vi "Write Config Files.vi"(8 "error in (no error)":errorcluster, 10 "Accessors:Config Session":T1) -> (0 "error out":errorcluster)   [LabVIEW 2015, in "Controller.lvlib" / "Controller.lvclass"]
doc: "Write the configuration files to the drives that we are writing to. This will prevent unnecessary loss of data in case of something breaking or a change in the configuration file."
uses:
  Controller.lvclass
  <vilib>/MSR Consulting, LLC/ESF/Typedefs/Session Handle.ctl
  <vilib>/MSR Consulting, LLC/ESF/Session - Root.lvclass
  reusable/Session APIs/File Access/Config Data/Config Data.lvclass
  reusable/Session APIs/File Access/Config Data/Config Data.lvclass/Config Data.ctl
  reusable/Session APIs/File Access/Config Data/Accessors/Read Ref.vi
  reusable/Session APIs/File Access/Config Data/Accessors/Read Cfg Path.vi
  <vilib>/Utility/config.llb/Read Key (Path).vi
  <vilib>/Utility/config.llb/NI_LVConfig.lvlib
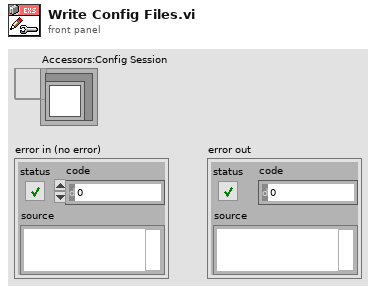
[diagram p1: front panel]
types:
  T1 = typedef "Session - Root.lvclass/Session Handle.ctl" = refnum<data-value>
  T2 = typedef "NI_LVConfig.lvlib/Config Data RefNum.ctl" = refnum<k1>
  T3 = typedef "LVDateTimeRec.ctl" = cluster{"fractional second":dbl, "second":i32, "minute":i32, "hour":i32, "day of month":i32, "month":i32, "year":i32, "day of week":i32, "day of year":i32, "DST":i32}
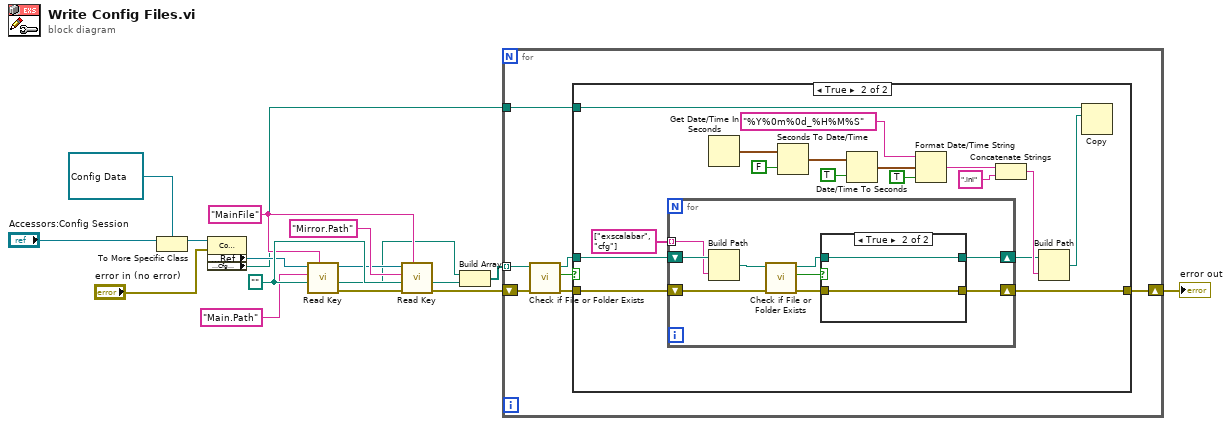
[diagram p0: block diagram]
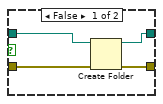
[diagram p3: hidden frame]
diagram:
  w17 = path ""
  w13 = "MainFile" ("section")
  n1 = To More Specific Class(target class=refnum<data-value> refnum, reference="Accessors:Config Session") -> (specific class reference=w11:refnum<data-value>)  [unwired: 1 in, 1 out]
  n2 = property class="Config Data"(reference=w11, error in="error in (no error)") -> ("Accessors:Ref"=w8:T2, "Accessors:Cfg Path"=w6:path)  [unwired: 2 out]
  n3 = call-poly <vilib>:"Read Key.vi"("section"=w13, "default value"=w17, "key"="Main.Path", "refnum"=w8) -> ("error out"=w15:errorcluster, "value"=w3:path, "refnum out"=w12:T2)  [unwired: 4 in, 1 out]
  n4 = call-poly <vilib>:"Read Key.vi"("section"=w13, "error in (no error)"=w15, "default value"=w17, "key"="Mirror.Path", "refnum"=w12) -> ("error out"=w5:errorcluster, "value"=w2:path)  [unwired: 3 in, 2 out]
  n5 = Build Array(w3, w2) -> (w1:path[])
  n6 = for {
    tunnel: w1 -> [w22] mode=indexing
    tunnel: w6 -> [w21]
    shift-right: [w18] -> w4
    shift-left: w5 -> [w20]
    n7 = call <vilib>:"Check if File or Folder Exists.vi"("error in (no error)"=w20, "path"=w22) -> ("error out"=w19:errorcluster, "file or folder exists?"=w23:bool, "dup path"=w24:path)  [unwired: 7 in]
    n8 = case shown="True" w23 {
      tunnel: w24 -> [_ w42]
      tunnel: w21 -> [_ w30]
      tunnel: w19 -> [w25 w29]
      tunnel: [w25 w28] -> w18
      frame False {
      }
      frame True {
        n9 = for {
          tunnel: string[] ["exscalabar", "cfg"] -> [w49] mode=indexing
          shift-right: [w45] -> w27
          shift-left: w42 -> [w50]
          shift-right: [w43] -> w28
          shift-left: w29 -> [w48]
          n10 = Build Path(base path=w50, name or relative path=w49) -> (appended path=w51:path)
          n11 = call <vilib>:"Check if File or Folder Exists.vi"("error in (no error)"=w48, "path"=w51) -> ("error out"=w44:errorcluster, "file or folder exists?"=w47:bool, "dup path"=w46:path)  [unwired: 7 in]
          n12 = case shown="True" w47 {
            tunnel: w46 -> [w55 w57]
            tunnel: [w54 w57] -> w45
            tunnel: w44 -> [w53 w56]
            tunnel: [w52 w56] -> w43
            frame False {
              n13 = Create Folder(path (use dialog)=w55, error in=w53) -> (created path=w54:path, error out=w52:errorcluster)  [unwired: 1 in, 1 out]
            }
            frame True {
            }
          }
        }
        n14 = Get Date/Time In Seconds() -> (seconds since 1Jan1904=w38:timestamp)
        n15 = Seconds To Date/Time(time stamp (now)=w38, to UTC (F)=FALSE) -> (date time rec=w35:T3)
        n16 = Date/Time To Seconds(1:TRUE ("is UTC (F)"), 2:w35) -> (0:w34:timestamp)
        n17 = Format Date/Time String(time format string (%c)="%Y%0m%0d_%H%M%S", seconds (now)=w34, UTC format=TRUE) -> (date/time string=w39:string)
        n18 = Concatenate Strings(w39, ".ini" ("string")) -> (w32:string)
        n19 = Build Path(base path=w27, name or relative path=w32) -> (appended path=w31:path)
        n20 = Copy(10:w31, 11:w30) -> ()  [unwired: 3 in, 3 out]
      }
    }
  }
  "error out" <- w4
